vi "LoadFileSettingControl.vi"(10 "This VI":refnum<vi>, 11 "MainMenu_In":refnum<vi>) -> ()   [LabVIEW 2013]
panel:
  out "error out":errorcluster
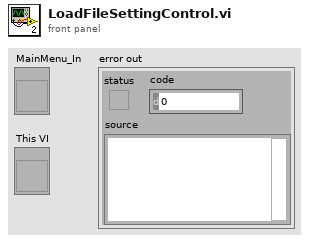
[diagram p1: front panel]
types:
  T1 = cluster{"Measurement":bool, "Save Data":bool, "LoadSetting":bool, "Save setting":bool, "Reset setting":bool, "Exit":bool}
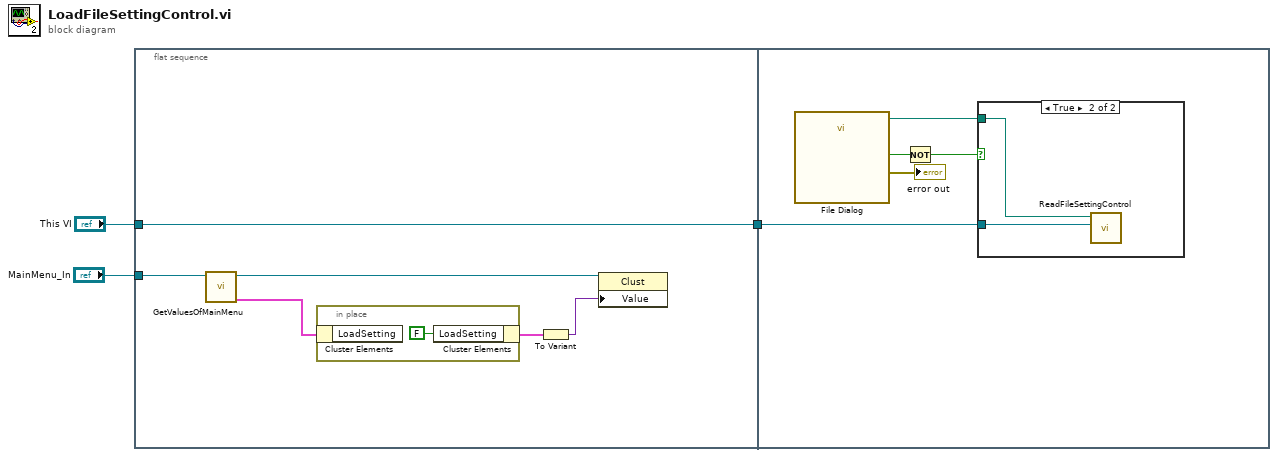
[diagram p0: block diagram]
diagram:
  n1 = flat-sequence {
    tunnel: "This VI" -> [w9]
    tunnel: [w9] -> w2
    tunnel: "MainMenu_In" -> [w8]
    tunnel: w2 -> [w11]
    frame #0 {
      n2 = call "GetValuesOfMainMenu.vi"("MainMenu_In"=w8) -> ("ValuesOfMainMenu"=w7:T1, "MainMenu_Out"=w6:refnum<vi>)  [unwired: 9 in]
      n3 = in-place {
        n4 = in-place-cluster #1(w7) -> ()  [unwired: 1 out]
        n5 = in-place-cluster #1("LoadSetting"=FALSE) -> (w5:T1)
      }
      n6 = To Variant(anything=w5) -> (Variant=w4:variant)
      n7 = property class="Clust"(reference=w6, "Value"=w4) -> ()  [unwired: 1 in, 2 out]
    }
    frame #1 {
      n8 = call "File Dialog"() -> ("selected path"=w15:path, "cancelled"=w12:bool, "error out"=→"error out":errorcluster)  [unwired: 12 in, 1 out]
      n9 = Not(x=w12) -> (.not. x?=w14:bool)
      n10 = case shown="True" w14 {
        tunnel: w11 -> [_ w17]
        tunnel: w15 -> [_ w16]
        frame False {
        }
        frame True {
          n11 = call "ReadFileSettingControl.vi"("ThisVI_In"=w17, "Path to was selected by user"=w16) -> ()  [unwired: 9 in, 1 out]
        }
      }
    }
  }
